vi "PH_Sequencer.get 4Q Position by Instance Name.vi"(0 "VI in":refnum<vi>, 2 "Wanted 4Q Instance":T1, 5 "error in":errorcluster) -> (14 "VI out":refnum<vi>, 15 "index of element":i32, 16 "Instancename":string, 17 "linked":bool, 18 "Current Position":T2 items=["unknown", "Position I", "Position II", "Position III", "Position IV", "moving"], 19 "error out":errorcluster)   [LabVIEW 2014, in "PH_Sequencer.lvlib"]
uses:
  PH_Sequencer.lvlib
  PH_Motion/PH_4_Pos_Selector/PH_4_Pos_Selector.Position Selector.ctl
  PH_Beamline/PH_Beamline.6P 4 Pos Selector Instances.ctl
  PH_Motion/PH_4_Pos_Selector/PH_4_Pos_Selector.lvlib
  PH_Beamline/PH_Beamline.lvlib
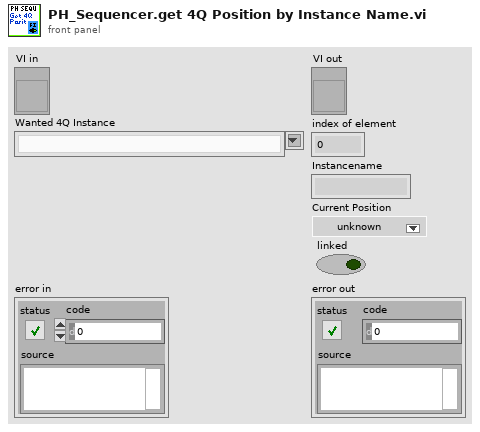
[diagram p1: front panel]
types:
  T1 = typedef "PH_Beamline.lvlib/PH_Beamline.6P 4 Pos Selector Instances.ctl" = string
  T2 = typedef "PH_4_Pos_Selector.lvlib/PH_4_Pos_Selector.Position Selector.ctl" = u16
  T3 = typedef "PH_Sequencer.lvlib/PH_Sequencer.i attribute.ctl" = cluster{"GUI Refs":cluster{"Main Off":refnum<vi>, "Fire":refnum<vi>, "Status":refnum<vi>, "Ready":refnum<vi>, "Waiting Time":refnum<vi>, "Timeout":refnum<vi>, "PPMA Ready":refnum<vi>, "Sequencer SM State":refnum<vi>, "PPPA Ready":refnum<vi>, "Calorimeter":refnum<vi>, "Beamline Ready":refnum<vi>, "Clear Beamline":refnum<vi>, "Linkage PPMA Rods":refnum<vi>, "Linkage Current PA":refnum<vi>, "Linkage Current MA":refnum<vi>, "Timing Ready":refnum<vi>, "State Timing":refnum<vi>, "Force Timing":refnum<vi>, "PSDB Shot Comment":refnum<vi>, "State PA Backreflection":refnum<vi>, "Beamline Z6 Ready":refnum<vi>, "Clear Z6 Beamline":refnum<vi>, "Sequence length":refnum<vi>, "Timing Mode":refnum<vi>, "Slow Trigger Settings":refnum<vi>, "Experiment Description":refnum<vi>, "State PSDB":refnum<vi>, "PSDB Ready":refnum<vi>, "Set PSDB Settings":refnum<vi>, "Get PSDB Info":refnum<vi>, "Take Snapshot":refnum<vi>, "Shottype":refnum<vi>, "Experiment":refnum<vi>, "Phase Frontends":refnum<vi>, "PP 45mm PILC in use":refnum<vi>}, "Status Info":cluster{"Machine Status":T4, "WaitingTime":i32, "Timeout":bool}, "Readyness":cluster{"Ready to shot":bool, "PPMA Ready":bool, "PPPA Ready":bool, "BL Ready":bool, "Timing Ready":bool, "BL Z6 Ready":bool, "PSDBReady":bool}, "Instancenames":cluster{"PPMA Rods":string, "PP Current Meas":string, "PH Beamline Chief":string, "PA Backrefl Meas":string, "Z6 Beamline Chief":string}, "Data to read":bool, "Calorimeter":cluster{"Instancename":string, "On":bool, "linked":bool}, "Linkage":cluster{"PPMA Rods":bool, "PP Current Meas":bool, "PHELIX Beamline Chief":bool, "PA Backrefl Meas":bool, "Z6 Beamline Chief":bool}, "Timing":cluster{"Instance":string, "linked":bool, "Status":T4, "Timing Mode":T5, "Slow Trigger Settings":T6, "Info available":cluster{"ext SlowTrigger":bool, "T2":bool, "Mode":bool, "Delay Slow Trigger":bool, "Phase FEs":bool}, "FE Phase":T7}, "Service ID R2S":i32, "PSDB":cluster{"Controller Instance":string, "Controller Status":T4, "Controller linked":bool, "Settings acknowledged":bool, "Current Experiment ID":i16, "Current Shot Type":i16, "Current Comment":string, "Remember Settings":bool, "Write 2 early":bool}, "PSDB Data":cluster{"Main Off?":bool, "Sequence Length":dbl, "Sequence startet":timestamp}, "6P 4Q Positions":cluster{"Instancename":string, "linked":bool, "Position":T2}[], "PUs":T8[]}
  T4 = typedef "PH_StatusHandler.lvlib/PH_StatusHandler.Status.ctl" = i16
  T5 = typedef "PH_Timing.lvlib/PH_Timing.Timing Mode.ctl" = cluster{"T2":i16, "Modeselector":enum32{"10 Hz", "0.5 Hz", "Shot"}}
  T6 = typedef "PH_Timing.lvlib/PH_Timing.Slow Trigger Settings.ctl" = cluster{"Delay":dbl, "externally triggered?":bool}
  T7 = typedef "PH_Timing.lvlib/PH_Timing.Phase FEs.ctl" = cluster{"Phase":dbl}
  T8 = typedef "PH_Sequencer.lvlib/PH_Sequencer.Head.ctl" = cluster{"PowerUnit":T9, "GUI Ref":refnum<vi>, "Information":T10, "linked?":bool, "GUI Ref Current Voltage":refnum<vi>}
  T9 = typedef "PH_PP_Common.lvlib/PH_PP_Common.PUs.ctl" = enum16{"no Info", "PA-19mm-1", "PA-19mm-2", "PA-45mm-PILC", "PA-45mm-MAIN", "MA-PU-1", "MA-PU-2", "MA-PU-3", "MA-PU-4", "MA-PU-5", "MA-PU-6", "MA-FR", "MA-PILC", "PA-45mm-DP"}
  T10 = typedef "PH_Sequencer.lvlib/PH_Sequencer.PU Information.ctl" = cluster{"State":T4, "Waiting Time [s]":dbl, "PU State SM":T11, "PU Timeout SM":T11}
  T11 = typedef "PH_PowerUnit_BaseClass.lvlib/PH_PowerUnit_BaseClass.SM States.ctl" = enum16{".", "Stand by", "Switch PU on", "Configure", "Set Default Voltage", "Set STANDBY", "Set READY", "Wait for Shot Cmd", "Open Dump Rods", "Open Ross Relais", "Close Ross Relais", "Switch PSU on", "Switch PSU off", "Charge", "Switch GD Channel on", "Close Dump Rods", "Rods-TO", "RR-TO", "PSU-TO", "Trigger-TO"}
  T12 = cluster{"Instancename":string, "linked":bool, "Position":T2}[]
  T13 = cluster{"Instancename":string, "linked":bool, "Position":T2}
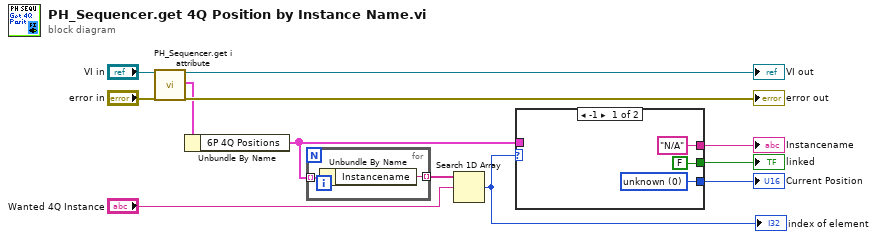
[diagram p0: block diagram]
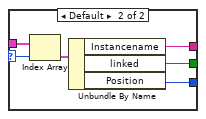
[diagram p2: hidden frame]
diagram:
  n1 = call "PH_Sequencer.get i attribute.vi"("i ref in"="VI in", "error in (no error)"="error in") -> ("i ref out"=→"VI out":refnum<vi>, "i attribute"=w5:T3, "error out"=→"error out":errorcluster)  [unwired: 15 in]
  n2 = Unbundle By Name(w5) -> ("6P 4Q Positions"=w4:T12)
  n3 = for {
    tunnel: w4 -> [w14] mode=indexing
    tunnel: [w13] -> w3 mode=indexing
    n4 = Unbundle By Name(w14) -> ("Instancename"=w13:string)
  }
  n5 = Search 1D Array(1D array=w3, element="Wanted 4Q Instance") -> (index of element=w1:i32)  [unwired: 1 in]
  "index of element" <- w1
  n6 = case shown="-1" w1 {
    selector: w1 -> [_ w18]
    tunnel: [w15 w23] -> w10
    tunnel: ["N/A" ("Instancename") w22] -> w9
    tunnel: [FALSE ("linked") w21] -> w8
    tunnel: w4 -> [_ w19]
    frame -1 {
      w15 = T2 0 items=["unknown", "Position I", "Position II", "Position III", "Position IV", "moving"] ("Position")
    }
    frame Default {
      n7 = Index Array(array=w19, index=w18) -> (element=w20:T13)
      n8 = Unbundle By Name(w20) -> ("Instancename"=w22:string, "linked"=w21:bool, "Position"=w23:T2)
    }
  }
  "Current Position" <- w10
  "Instancename" <- w9
  "linked" <- w8
